vi "Begin.vi"(8 "error in":errorcluster) -> (0 "error out":errorcluster)   [LabVIEW 2020]
doc: "Called before other user functions, this VI is expected to open initial I/O refnums, load in file data, and do all program initialization. Notice that the <B>error out</B> terminal is simply used for data flow. Wiring it to other structures or subVIs ensures that this VI runs first."
uses:
  <vilib>/Rock Robotics/WPI/DriverStation/WPI_DriverStationRobotMode2.ctl
  <vilib>/Rock Robotics/WPI/Joystick/WPI_JoystickDeviceEnum.ctl
  <vilib>/Rock Robotics/WPI/Solenoid/WPI_SolenoidChannel.ctl
  <vilib>/Rock Robotics/SystemInterfaces/DIO/FPGA_DIOPWMChannel.ctl
  <vilib>/Rock Robotics/WPI/SafetyOutput/WPI_SafetyOutputConfigMenu.ctl
  Robot Global Data.vi
  <vilib>/Rock Robotics/Network Tables/NT Write String Array.vi
  <vilib>/Rock Robotics/WPI/Solenoid/WPI_SolenoidOpenDouble.vi
  <vilib>/Rock Robotics/WPI/MotorControl/WPI_MotorControlOpen VictorSP.vi
  <vilib>/Rock Robotics/WPI/RobotDrive/WPI_RobotDriveOpen2MotorWithExistingMotors.vi
  <vilib>/Rock Robotics/WPI/Utilities/WPI_GetSetVariantRefNum.vi
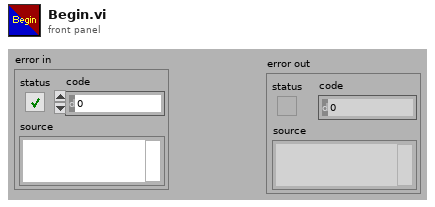
[diagram p1: front panel]
types:
  T1 = typedef "WPI_SafetyOutputConfigMenu.ctl" = enum16{"Enable", "Disable"}
  T2 = typedef "FPGA_DIOPWMChannel.ctl" = enum8{"PWM 0", "PWM 1", "PWM 2", "PWM 3", "PWM 4", "PWM 5", "PWM 6", "PWM 7", "PWM 8", "PWM 9", "PWM MXP 0", "PWM MXP 1", "PWM MXP 2", "PWM MXP 3", "PWM MXP 4", "PWM MXP 5", "PWM MXP 6", "PWM MXP 7", "PWM MXP 8", "PWM MXP 9", "Invalid"}
  T3 = typedef "WPI_JoystickDeviceEnum.ctl" = enum16{"USB 0", "USB 1", "USB 2", "USB 3", "USB 4", "USB 5"}
  T4 = typedef "WPI_SolenoidChannel.ctl" = enum8{"Solenoid 0", "Solenoid 1", "Solenoid 2", "Solenoid 3", "Solenoid 4", "Solenoid 5", "Solenoid 6", "Solenoid 7", "Solenoid 8", "Solenoid 9", "Solenoid 10", "Solenoid 11", "Solenoid 12", "Solenoid 13", "Solenoid 14", "Solenoid 15", "Invalid"}
  T5 = typedef "WPI_DriverStationRobotMode2.ctl" = enum16{"Autonomous Disabled", "Autonomous Enabled", "Teleop Disabled", "Teleop Enabled", "Disconnected", "Finish", "Test Disabled", "Test Enabled", "Emergency Stopped"}
  T6 = typedef "WPI_MotorControlDeviceRef.ctl" = cluster{"DeviceStatus":errorcluster, "Type":T7, "PWM":cluster{"PWM Channel":T2, "DeadBand":T8}, "CAN":cluster{"Device Number":u8, "SetOutput VI Ref":variant, "GetOutput VI Ref":variant, "Enable VI Ref":variant, "Disable VI Ref":variant, "Data":variant}, "Invert":bool, "DIO PWM":cluster{"PWM \"Enable\" Channel":T2, "DIOChannel":T9, "PWM Rate":dbl}}
  T7 = typedef "WPI_MotorControlType.ctl" = enum16{"PWM", "CAN", "DIO PWM"}
  T8 = typedef "WPI_PWMDeadband.ctl" = cluster{"Name":string, "maxPositivePwm":i32, "minPositivePwm":i32, "centerPwm":i32, "maxNegativePwm":i32, "minNegativePwm":i32, "angularRange":u16}
  T9 = typedef "FPGA_DIOChannel.ctl" = enum8{"DIO 0", "DIO 1", "DIO 2", "DIO 3", "DIO 4", "DIO 5", "DIO 6", "DIO 7", "DIO 8", "DIO 9", "DIO MXP 0", "DIO MXP 1", "DIO MXP 2", "DIO MXP 3", "DIO MXP 4", "DIO MXP 5", "DIO MXP 6", "DIO MXP 7", "DIO MXP 8", "DIO MXP 9", "DIO MXP 10", "DIO MXP 11", "DIO MXP 12", "DIO MXP 13", "DIO MXP 14", "DIO MXP 15", "SPI Port CS1", "SPI Port CS2", "SPI Port CS3", "SPI Port MISO", "SPI Port MOSI", "Invalid"}
  T10 = typedef "WPI_RobotDriveDevRef.ctl" = cluster{"DevStatus":errorcluster, "Motors[]":T6[], "Square Inputs":bool, "Max Output":dbl}
  T11 = typedef "WPI_JoystickDevRef.ctl" = cluster{"Device":T3}
  T12 = typedef "WPI_CompressorDevRef.ctl" = cluster{"DevStatus":errorcluster, "Pneumatics Control Module":u8}
  T13 = typedef "WPI_SolenoidDevRef.ctl" = cluster{"DevStatus":errorcluster, "Pneumatics Control Module":u8, "Forward Solenoid Channel":T4, "Reverse Solenoid Channel":T4}
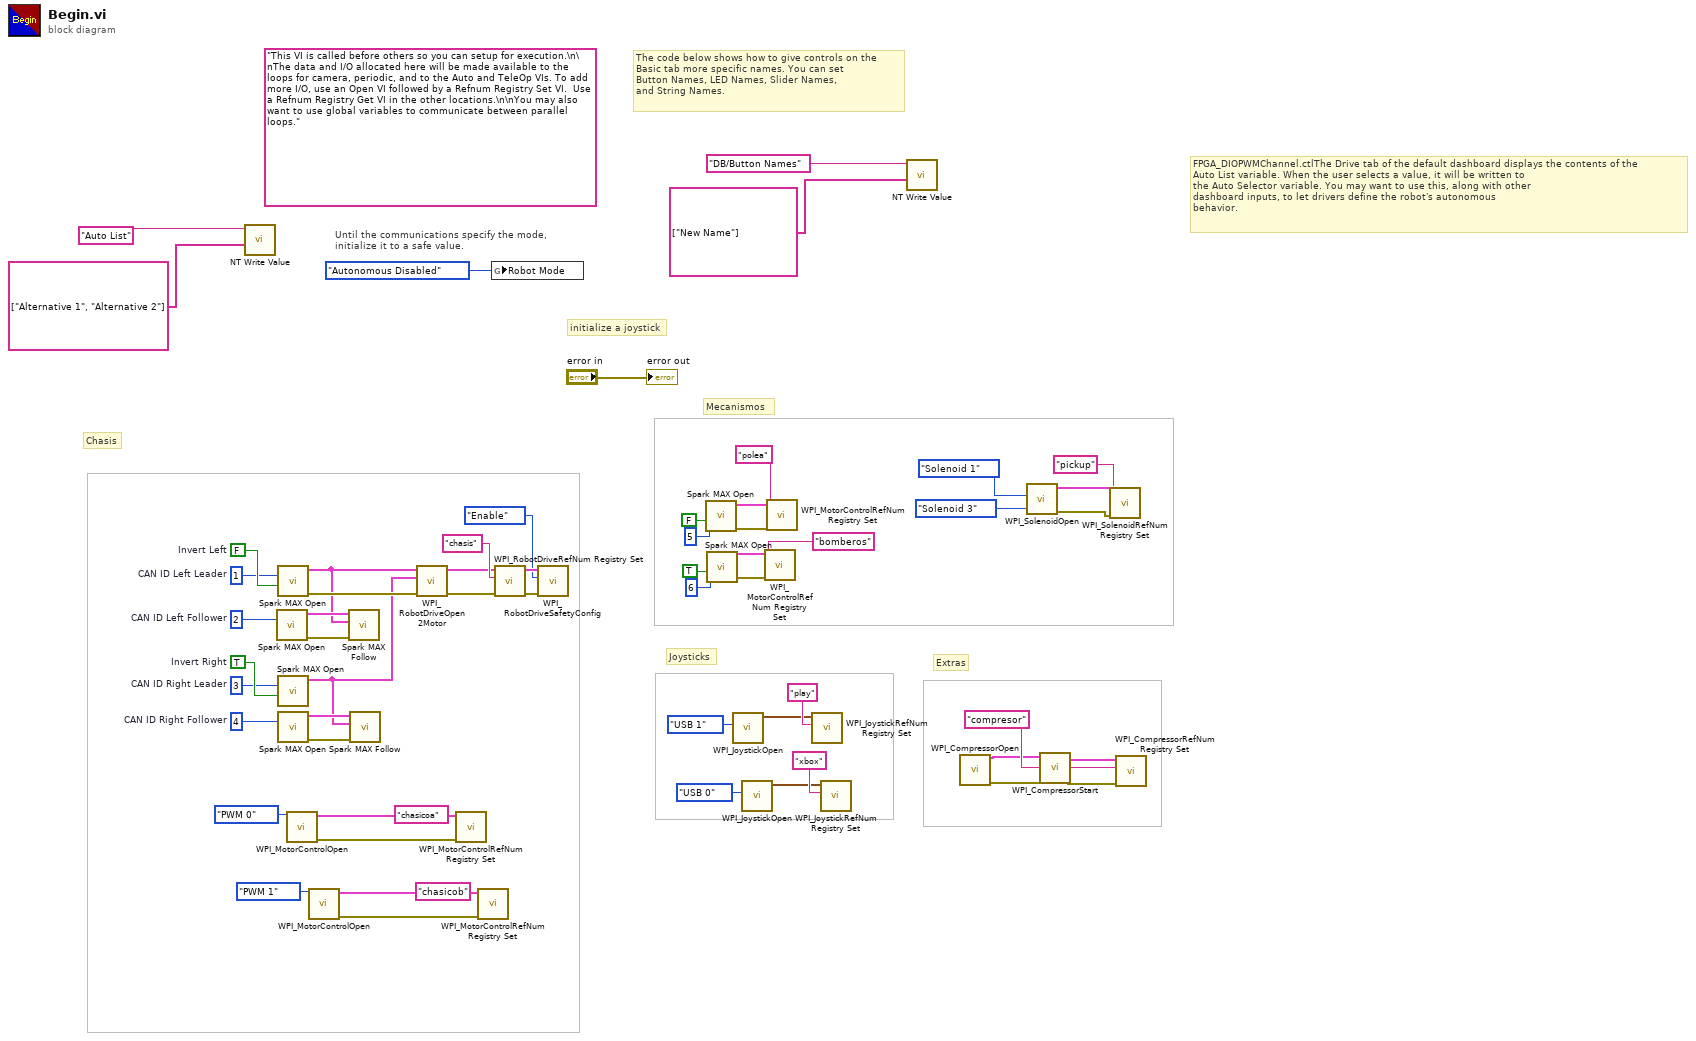
[diagram p0: block diagram]
diagram:
  w19 = FALSE  # Invert Left
  w18 = TRUE  # Invert Right
  w10 = u8 3  # CAN ID Right Leader
  w11 = u8 4  # CAN ID Right Follower
  w3 = u8 1  # CAN ID Left Leader
  w2 = u8 2  # CAN ID Left Follower
  (unwired) "This VI is called before others so you can setup for execution.\n\nThe data and I/O allocated here will be made available to the loops for camera, periodic, and to the Auto and TeleOp VIs. To add more I/O, use an Open VI followed by a Refnum Registry Set VI.  Use a Refnum Registry Get VI in the other locations.\n\nYou may also want to use global variables to communicate between parallel loops."
  # "Extras"
  # "Joysticks"
  # "Mecanismos"
  # "Chasis"
  # "FPGA_DIOPWMChannel.ctlThe Drive tab of the default dashboard displays the contents of the\nAuto List variable. When the user selects a value, it will be written to\nthe Auto Selector variable. You may want to use this, along with other\ndashboard inputs, to let drivers define the robot's autonomous\nbehavior."
  # "The code below shows how to give controls on the\nBasic tab more specific names. You can set\nButton Names, LED Names, Slider Names,\nand String Names."
  # "initialize a joystick"
  # "Until the communications specify the mode,\ninitialize it to a safe value."
  n1 = call-poly <vilib>:"NT Write Value.vi"("String Array"=string[] ["Alternative 1", "Alternative 2"], "Name"="Auto List") -> ()  [unwired: 9 in, 1 out]
  n2 = call <vilib>:"Spark MAX Open.vi"("Device Number"=w2) -> ("error out"=w7:errorcluster, "MotorControlDeviceRef"=w6:T6)  [unwired: 9 in]
  n3 = call <vilib>:"Spark MAX Open.vi"("Invert"=w19, "Device Number"=w3) -> ("error out"=w5:errorcluster, "MotorControlDeviceRef"=w4:T6)  [unwired: 8 in]
  n4 = call <vilib>:"Spark MAX Open.vi"("Invert"=w18, "Device Number"=w10) -> ("MotorControlDeviceRef"=w1:T6)  [unwired: 8 in, 1 out]
  n5 = call <vilib>:"Spark MAX Open.vi"("Device Number"=w11) -> ("error out"=w8:errorcluster, "MotorControlDeviceRef"=w9:T6)  [unwired: 9 in]
  n6 = call-poly <vilib>:"WPI_MotorControlOpen.vi"("PWM Channel"=FPGA_DIOPWMChannel."PWM 0") -> ("error out"=w35:errorcluster, "MotorControlDeviceRef"=w36:T6)  [unwired: 9 in]
  n7 = call-poly <vilib>:"WPI_MotorControlOpen.vi"("PWM Channel"=FPGA_DIOPWMChannel."PWM 1") -> ("error out"=w31:errorcluster, "MotorControlDeviceRef"=w32:T6)  [unwired: 9 in]
  n8 = call <vilib>:"Spark MAX Follow.vi"("error in (no error)"=w7, "Master Controller"=w4, "MotorControlDeviceRef"=w6) -> ()  [unwired: 7 in, 2 out]
  n9 = call <vilib>:"Spark MAX Follow.vi"("error in (no error)"=w8, "Master Controller"=w1, "MotorControlDeviceRef"=w9) -> ()  [unwired: 7 in, 2 out]
  n10 = call-poly <vilib>:"WPI_RobotDriveOpen2Motor.vi"("error in (no error)"=w5, "Right Motor Dev Ref"=w1, "Left Motor Dev Ref"=w4) -> ("error out"=w14:errorcluster, "RobotDriveDevRef"=w12:T10)  [unwired: 7 in]
  n11 = call <vilib>:"WPI_MotorControlRefNum Registry Set.vi"("error in (no error)"=w35, "refnum name"="chasicoa", "MotorControlDevRef"=w36) -> ()  [unwired: 7 in, 2 out]
  n12 = call <vilib>:"WPI_MotorControlRefNum Registry Set.vi"("error in (no error)"=w31, "refnum name"="chasicob", "MotorControlDevRef"=w32) -> ()  [unwired: 7 in, 2 out]
  n13 = global write "Robot Global Data.vi" "Robot Mode"(WPI_DriverStationRobotMode2."Autonomous Disabled" ("Robot Mode")) -> ()
  n14 = call <vilib>:"WPI_RobotDriveRefNum Registry Set.vi"("error in (no error)"=w14, "refnum name"="chasis", "RobotDriveDevRef"=w12) -> ("error out"=w17:errorcluster, "RobotDriveDevRef"=w16:T10)  [unwired: 7 in]
  n15 = call <vilib>:"WPI_RobotDriveSafetyConfig.vi"("error in (no error)"=w17, "mode"=WPI_SafetyOutputConfigMenu."Enable", "RobotDriveDevRef"=w16) -> ()  [unwired: 7 in, 2 out]
  n16 = call <vilib>:"Spark MAX Open.vi"("Invert"=FALSE, "Device Number"=u8 5) -> ("error out"=w28:errorcluster, "MotorControlDeviceRef"=w29:T6)  [unwired: 8 in]
  n17 = call <vilib>:"Spark MAX Open.vi"("Invert"=TRUE, "Device Number"=u8 6) -> ("error out"=w26:errorcluster, "MotorControlDeviceRef"=w27:T6)  [unwired: 8 in]
  n18 = call <vilib>:"WPI_JoystickOpen.vi"("JoystickDevice"=WPI_JoystickDeviceEnum."USB 1") -> ("JoystickDevRef"=w44:T11)  [unwired: 10 in]
  n19 = call <vilib>:"WPI_JoystickOpen.vi"("JoystickDevice"=WPI_JoystickDeviceEnum."USB 0") -> ("JoystickDevRef"=w57:T11)  [unwired: 10 in]
  n20 = call <vilib>:"WPI_MotorControlRefNum Registry Set.vi"("error in (no error)"=w26, "refnum name"="bomberos", "MotorControlDevRef"=w27) -> ()  [unwired: 7 in, 2 out]
  n21 = call <vilib>:"WPI_MotorControlRefNum Registry Set.vi"("error in (no error)"=w28, "refnum name"="polea", "MotorControlDevRef"=w29) -> ()  [unwired: 7 in, 2 out]
  n22 = call <vilib>:"WPI_JoystickRefNum Registry Set.vi"("refnum name"="play", "JoystickDevRef"=w44) -> ()  [unwired: 8 in, 2 out]
  n23 = call <vilib>:"WPI_JoystickRefNum Registry Set.vi"("refnum name"="xbox", "JoystickDevRef"=w57) -> ()  [unwired: 8 in, 2 out]
  n24 = call-poly <vilib>:"NT Write Value.vi"("String Array"=string[] ["New Name"], "Name"="DB/Button Names") -> ()  [unwired: 9 in, 1 out]
  n25 = call <vilib>:"WPI_CompressorOpen.vi"() -> ("CompressorDevRef"=w41:T12, "error out"=w40:errorcluster)  [unwired: 14 in]
  n26 = call-poly <vilib>:"WPI_SolenoidOpen.vi"("Reverse Solenoid Channel"=WPI_SolenoidChannel."Solenoid 3", "Forward Solenoid Channel"=WPI_SolenoidChannel."Solenoid 1") -> ("error out"=w49:errorcluster, "SolenoidDevRef"=w50:T13)  [unwired: 8 in]
  n27 = call <vilib>:"WPI_CompressorStart.vi"("error in (no error)"=w40, "CompressorDevRef"=w41) -> ("error out"=w38:errorcluster, "CompressorDevRef"=w39:T12)  [unwired: 8 in]
  n28 = call <vilib>:"WPI_SolenoidRefNum Registry Set.vi"("error in (no error)"=w49, "refnum name"="pickup", "SolenoidDevRef"=w50) -> ()  [unwired: 7 in, 2 out]
  n29 = call <vilib>:"WPI_CompressorRefNum Registry Set.vi"("error in (no error)"=w38, "refnum name"="compresor", "CompressorDevRef"=w39) -> ()  [unwired: 7 in, 2 out]
  "error out" <- "error in"
